vi "Pololu.Mgr - Set Position in Degrees.vi"(6 "Ignore Stops":bool, 8 "error in (no error)":errorcluster, 9 "Pos(Deg)":dbl, 10 "Channel":u8, 11 "PololuCtrl in":refnum<class "PololuCtrl.lvclass">) -> (0 "error out":errorcluster, 1 "Actual Pos(us)":dbl, 2 "Actual Pos(Deg)":dbl, 3 "PololuCtrl out":refnum<class "PololuCtrl.lvclass">)   [LabVIEW 2018, in "PololuCtrl.lvclass"]
uses:
  PololuCtrl.lvclass
  PololuCtrl.lvclass/PololuCtrl.ctl
  SubVIs/Pololu.Message Byte Defs.ctl
  Serial Port/Class/SerialPort.lvclass
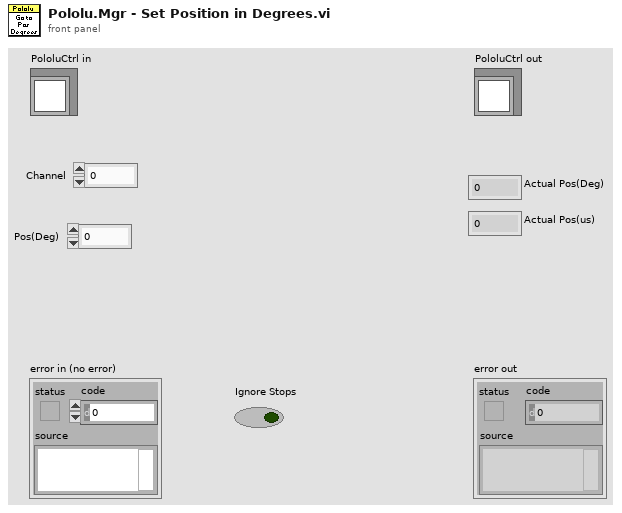
[diagram p1: front panel]
types:
  T1 = typedef "Pololu.Device Config.ctl" = cluster{"Chan":u8, "Accel":u16, "Speed":u16, "Positions":dbl[], "Range Info":T2}
  T2 = typedef "Pololu.Device Range Config.ctl" = cluster{"Min us":dbl, "Max us":dbl, "Min deg":dbl, "Max deg":dbl, "LStopDeg":dbl, "UStopDeg":dbl}
  T3 = cluster{"Channel":u8, "Pos":u16, "Response":u16, "Bytes":u8[], "Query":bool}
  T4 = typedef "Pololu.Message Byte Defs.ctl" = u8
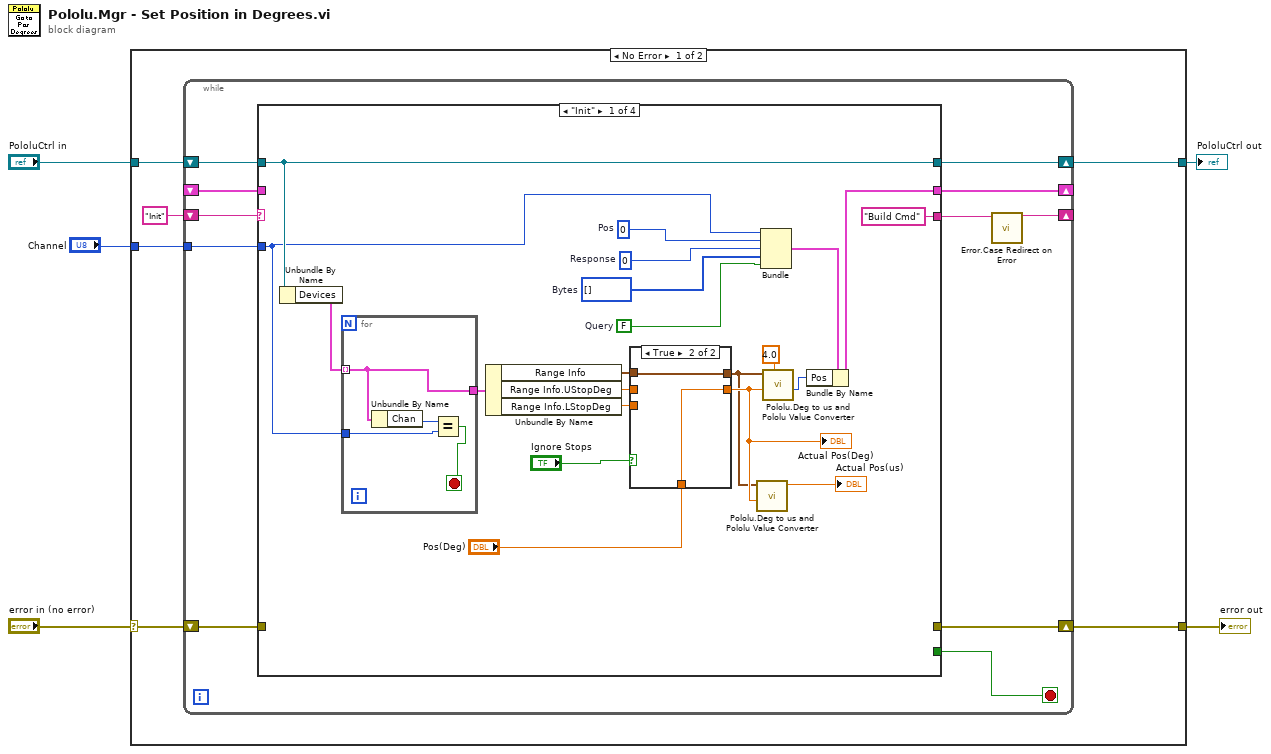
[diagram p0: block diagram]
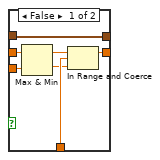
[diagram p2: hidden frame]
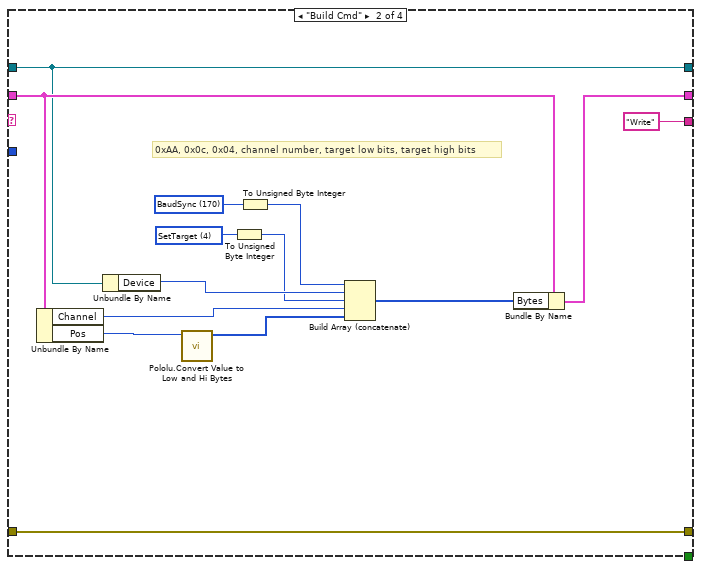
[diagram p3: hidden frame]
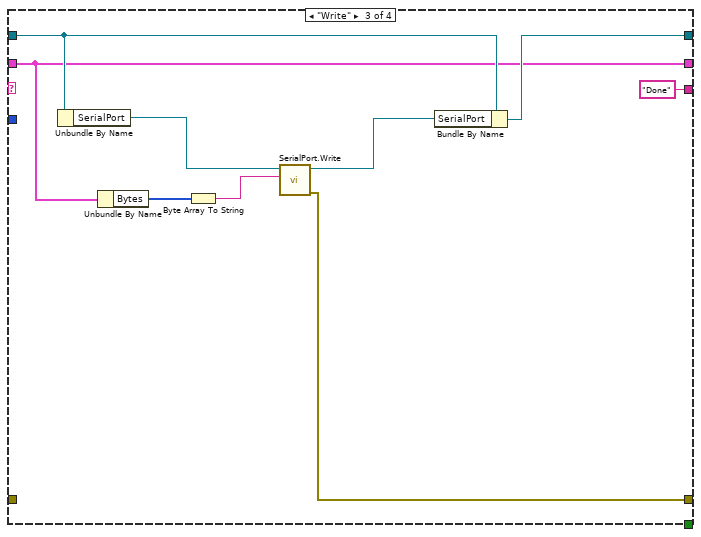
[diagram p4: hidden frame]
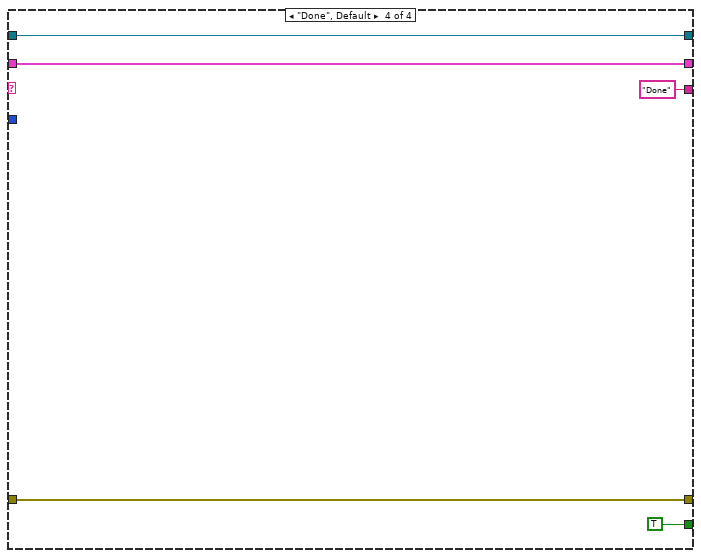
[diagram p5: hidden frame]
diagram:
  n1 = case shown="No Error" "error in (no error)" {
    selector: "error in (no error)" -> [w10 w86]
    tunnel: [w7 w86] -> w4
    tunnel: [w9 w85] -> w2
    tunnel: "PololuCtrl in" -> [w11 w85]
    tunnel: "Channel" -> [w6 _]
    frame No Error {
      n2 = while {
        shift-right: [w21] -> w9
        shift-left: w11 -> [w22]
        shift-right: [w14] -> w7
        shift-left: w10 -> [w15]
        shift-right: [w18] -> _
        shift-left: "Init" -> [w19]
        shift-right: [w16] -> _
        shift-left: _ -> [w20]
        tunnel: w6 -> [w12]
        stop <- w13 stop-if-true
        n3 = case shown="\"Init\"" w19 {
          tunnel: w22 -> [w38 w64 w76 w84]
          tunnel: [w38 w64 w77 w84] -> w21
          tunnel: w20 -> [_ w68 w72 w81]
          tunnel: ["Build Cmd" "Write" "Done" "Done"] -> w17
          tunnel: [w35 w69 w72 w81] -> w16
          tunnel: w15 -> [_ w70 _ w82]
          tunnel: [_ w70 w73 w82] -> w14
          tunnel: [_ _ _ TRUE] -> w13
          tunnel: w12 -> [w30 _ _ _]
          frame "Init" {
            w39 = u16 0  # Pos
            w42 = u16 0  # Response
            w40 = FALSE  # Query
            w41 = u8[] []  # Bytes
            n4 = Unbundle By Name(w38) -> ("Devices"=w37:T1[])
            n5 = for {
              tunnel: w37 -> [w56] mode=indexing
              tunnel: [w56] -> w34
              tunnel: w30 -> [w53]
              stop <- w54 stop-if-true
              n6 = Unbundle By Name(w56) -> ("Chan"=w55:u8)
              n7 = Equal?(x=w55, y=w53) -> (x = y?=w54:bool)
            }
            n8 = Unbundle By Name(w34) -> ("Range Info"=w25:T2, "Range Info.UStopDeg"=w27:dbl, "Range Info.LStopDeg"=w26:dbl)
            n9 = case shown="True" "Ignore Stops" {
              tunnel: "Pos(Deg)" -> [w50 w51]
              tunnel: [w49 w51] -> w29
              tunnel: w27 -> [w48 _]
              tunnel: w26 -> [w47 _]
              tunnel: w25 -> [w44 w52]
              tunnel: [w44 w52] -> w24
              frame False {
                n10 = Max & Min(x=w48, y=w47) -> (max(x,y)=w46:dbl, min(x,y)=w45:dbl)
                n11 = In Range and Coerce(upper limit=w46, x=w50, lower limit=w45) -> (coerced(x)=w49:dbl)  [unwired: 1 out]
              }
              frame True {
              }
            }
            "Actual Pos(Deg)" <- w29
            n12 = call "Pololu.Deg to us and Pololu Value Converter.vi"("Set Pos (Deg)"=w29, "Range Info"=w24) -> ("Cmd us"=→"Actual Pos(us)":dbl)  [unwired: 8 in, 1 out]
            n13 = Bundle("Channel"=w30, "Pos"=w39, "Response"=w42, "Bytes"=w41, "Query"=w40) -> (w36:T3)  [unwired: 1 in]
            n14 = call "Pololu.Deg to us and Pololu Value Converter.vi"("us to Units Mult"=4.0, "Set Pos (Deg)"=w29, "Range Info"=w24) -> ("Cmd units"=w32:u16)  [unwired: 7 in, 1 out]
            n15 = Bundle By Name(cluster=w36, "Pos"=w32) -> (w35:T3)
          }
          frame "Build Cmd" {
            w58 = T4 4 items=["BaudSync"=170, "SetTarget"=4, "Set Speed"=7, "Set Accel"=9, "Get Pos"=16, "Get MovStat"=19, "Get Errors"=33] ("Cmds")
            w59 = T4 170 items=["BaudSync"=170, "SetTarget"=4, "Set Speed"=7, "Set Accel"=9, "Get Pos"=16, "Get MovStat"=19, "Get Errors"=33] ("Cmds")
            # "0xAA, 0x0c, 0x04, channel number, target low bits, target high bits"
            n16 = Unbundle By Name(w68) -> ("Channel"=w67:u8, "Pos"=w66:u16)
            n17 = Unbundle By Name(w64) -> ("Device"=w63:u8)
            n18 = call "Pololu.Convert Value to Low and Hi Bytes.vi"("Value"=w66) -> ("Low_Hi Bytes"=w60:u8[])  [unwired: 10 in]
            n19 = To Unsigned Byte Integer(number=w58) -> (unsigned 8bit integer=w61:T4)
            n20 = To Unsigned Byte Integer(number=w59) -> (unsigned 8bit integer=w62:T4)
            n21 = Build Array (concatenate)(w62, w63, w61, w67, w60) -> (w65:T4[])
            n22 = Bundle By Name(cluster=w68, "Bytes"=w65) -> (w69:T3)
          }
          frame "Write" {
            n23 = Unbundle By Name(w76) -> ("SerialPort"=w75:refnum<class "SerialPort.lvclass">)
            n24 = Unbundle By Name(w72) -> ("Bytes"=w78:u8[])
            n25 = Byte Array To String(unsigned byte array=w78) -> (string=w71:string)
            n26 = call "SerialPort.Write.vi"("Data"=w71, "SerialPort in"=w75) -> ("error out"=w73:errorcluster, "SerialPort out"=w74:refnum<class "SerialPort.lvclass">)  [unwired: 6 in, 2 out]
            n27 = Bundle By Name(cluster=w76, "SerialPort"=w74) -> (w77:refnum<class "PololuCtrl.lvclass">)
          }
          frame "Done", Default {
          }
        }
        n28 = call "Error.Case Redirect on Error.vi"("Next Case"=w17) -> ("Next Case Out"=w18:string)  [unwired: 10 in]
      }
    }
    frame Error {
    }
  }
  "error out" <- w4
  "PololuCtrl out" <- w2
